vi "Set Attributes.vi"(8 "error in (no error)":errorcluster, 11 "For Loop Dialog in":refnum<class "For Loop Dialog.lvclass">) -> (0 "error out":errorcluster, 3 "For Loop Dialog out":refnum<class "For Loop Dialog.lvclass">)   [LabVIEW 2017, in "For Loop Dialog.lvclass"]
uses:
  For Loop Dialog.lvclass
  ITest Executive Builder Dialog/ITest Executive Builder Dialog.lvclass
  <vilib>/gpm_packages/@cs/test-executive/Source/Test Executive/TestExecutive Ref/TestExecutive Ref.lvclass
  59fac6ae-310b-4988-a921-2127789b6df3.vi
  58fb083d-74a7-4f00-8e06-222a9ebb18d7.vi
  C:/Users/jonmc/Documents/Git/Test Executive Builder/Source/Test Executive Builder Dialogs/ITest Executive Builder Dialog/ITest Executive Builder Dialog.lvclass
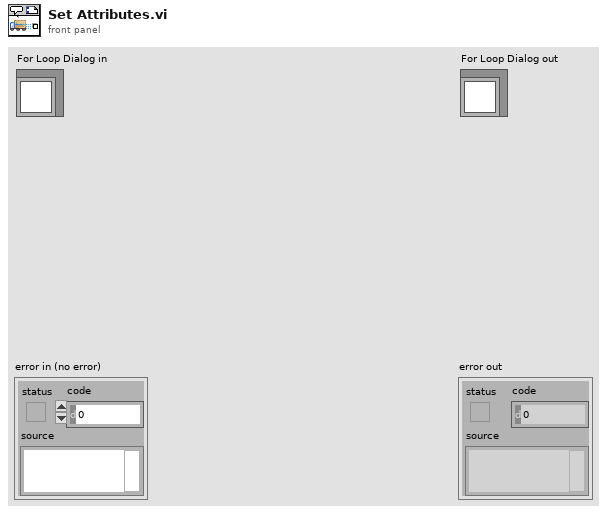
[diagram p1: front panel]
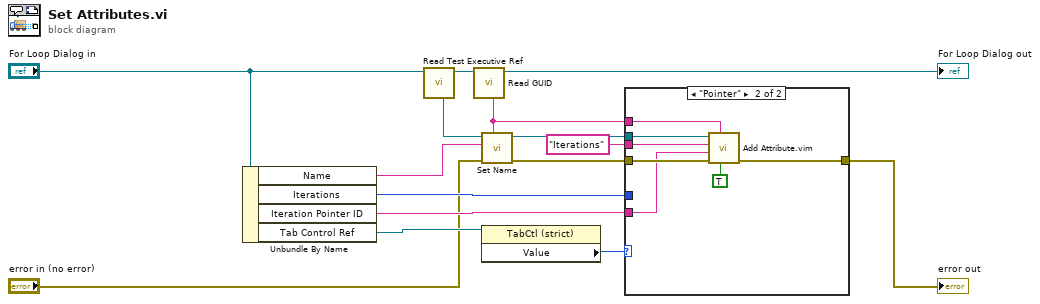
[diagram p0: block diagram]
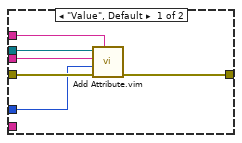
[diagram p2: hidden frame]
diagram:
  n1 = Unbundle By Name("For Loop Dialog in") -> ("Name"=w13:string, "Iterations"=w10:u32, "Iteration Pointer ID"=w9:string, "Tab Control Ref"=w12:refnum<vi>)
  n2 = call "Read Test Executive Ref.vi"("ITest Executive Builder Dialog in"="For Loop Dialog in") -> ("ITest Executive Builder Dialog out"=w15:refnum<class "For Loop Dialog.lvclass">, "Test Executive Ref"=w14:refnum<data-value>)  [unwired: 9 in]
  n3 = call "Read GUID.vi"("ITest Executive Builder Dialog in"=w15) -> ("ITest Executive Builder Dialog out"=→"For Loop Dialog out":refnum<class "For Loop Dialog.lvclass">, "GUID"=w7:string)  [unwired: 9 in]
  n4 = call <vilib>:"Set Name.vi"("Unique ID"=w7, "error in (no error)"="error in (no error)", "Name"=w13, "Test Executive Ref"=w14) -> ("error out"=w5:errorcluster, "Test Executive Ref out"=w8:refnum<data-value>)  [unwired: 6 in]
  n5 = property class="TabCtl (strict)"(reference=w12) -> ("Value"=w11:enum32{"Value", "Pointer"})  [unwired: 1 in, 2 out]
  n6 = case shown="\"Pointer\"" w11 {
    tunnel: w10 -> [w17 _]
    tunnel: w9 -> [_ w24]
    tunnel: w8 -> [w21 w28]
    tunnel: w7 -> [w20 w23]
    tunnel: "Iterations" -> [w19 w25]
    tunnel: w5 -> [w18 w27]
    tunnel: [w16 w22] -> w1
    frame "Value", Default {
      n7 = call "Add Attribute.vim"("ID"=w20, "error in (no error)"=w18, "Attribute"=w17, "Attribute Name"=w19, "Test Executive Ref"=w21) -> ("error out"=w16:errorcluster)  [unwired: 3 in, 3 out]
    }
    frame "Pointer" {
      n8 = call "Add Attribute.vim"("Pointer?"=TRUE, "ID"=w23, "error in (no error)"=w27, "Attribute"=w24, "Attribute Name"=w25, "Test Executive Ref"=w28) -> ("error out"=w22:errorcluster)  [unwired: 2 in, 3 out]
    }
  }
  "error out" <- w1
